vi "Configure Instrument.vi"(0 "VISA resource name":refnum<visa-resource-name>, 5 "Enable Keypad Lock (F: Off)":bool, 7 "Lock Code (123)":dbl=123.0, 9 "Remote Interface Mode (0:Local)":u16(ring) items=["Local", "Remote", "Remote with local lockout"], 11 "error in (no error)":errorcluster, 12 "Emulation Mode (0:None (335))":u16(ring) items=["None (335)", "331", "332"], 13 "PID Control Scaling (0:335 (Temperature))":u16(ring) items=["335 (Temperature)", "331/332 (Sensor)"]) -> (4 "VISA resource name out":refnum<visa-resource-name>, 15 "error out":errorcluster)   [LabVIEW 2014, in "Lake Shore 335.lvlib"]
doc: "Configures various instrument settings. Parameters configured are;\n331/332 Emulation, Remote interface mode, and keypad lock out."
uses:
  Lake Shore 335.lvlib
  Instance           1 28Saved   Configure Instrument .vi
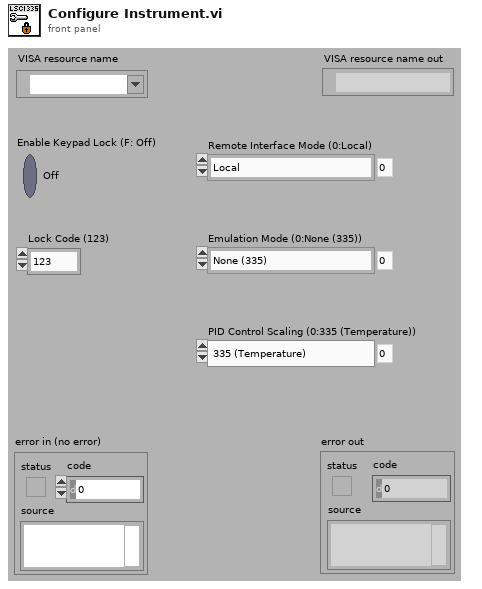
[diagram p1: front panel]
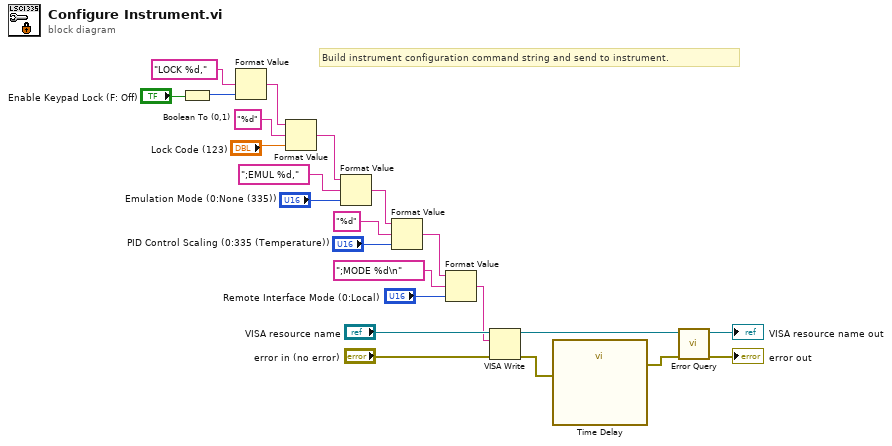
[diagram p0: block diagram]
diagram:
  # "Build instrument configuration command string and send to instrument."
  n1 = Boolean To (0,1)(Boolean="Enable Keypad Lock (F: Off)") -> (0, 1=w16:i16)
  n2 = Format Value(format string="LOCK %d,", value (0)=w16) -> (output string=w11:string)  [unwired: 1 in]
  n3 = Format Value(string ("")=w11, format string="%d", value (0)="Lock Code (123)") -> (output string=w2:string)
  n4 = Format Value(string ("")=w2, format string=";EMUL %d,", value (0)="Emulation Mode (0:None (335))") -> (output string=w4:string)
  n5 = Format Value(string ("")=w4, format string="%d", value (0)="PID Control Scaling (0:335 (Temperature))") -> (output string=w1:string)
  n6 = Format Value(string ("")=w1, format string=";MODE %d\n", value (0)="Remote Interface Mode (0:Local)") -> (output string=w3:string)
  n7 = VISA Write(VISA resource name="VISA resource name", write buffer=w3, error in (no error)="error in (no error)") -> (VISA resource name out=w21:refnum<visa-resource-name>, error out=w10:errorcluster)  [unwired: 1 out]
  n8 = call "Time Delay"("error in (no error)"=w10) -> ("error out"=w9:errorcluster)  [unwired: 10 in]
  n9 = call "Error Query.vi"("error in (no error)"=w9, "VISA resource name"=w21) -> ("error out"=→"error out":errorcluster, "VISA resource name out"=→"VISA resource name out":refnum<visa-resource-name>)  [unwired: 7 in, 1 out]
